vi "hse-configuration_GetAllKeysForSection.vi"(8 "error in (no error)":errorcluster, 10 "Section":string, 11 "hse-configuration in":refnum<class "hse-configuration.lvclass">) -> (0 "error out":errorcluster, 2 "Keys":string[](array[string]), 3 "hse-configuration out":refnum<class "hse-configuration.lvclass">)   [LabVIEW 2014, in "hse-configuration.lvclass"]
doc: "Reads the numeric configuration value (DOUBLE) identified by <b>section</b> and <b>key</b> from the configuration object\n\n____\nHAMPEL SOFTWARE ENGINEERING v0.12.0 (2018-09-13 18:21)"
uses:
  hse-configuration.lvclass
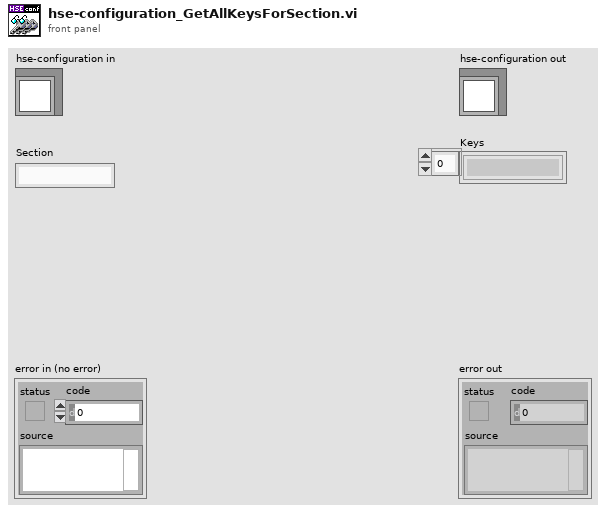
[diagram p1: front panel]
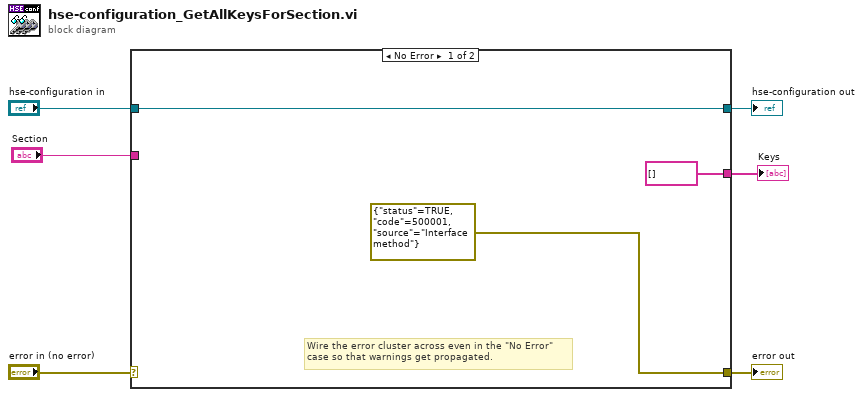
[diagram p0: block diagram]
diagram:
  n1 = case shown="No Error" "error in (no error)" {
    selector: "error in (no error)" -> [_ w11]
    tunnel: [errorcluster {"status"=TRUE, "code"=500001, "source"="Interface method"} ("error IO") w11] -> w5
    tunnel: [w9 w10] -> w3
    tunnel: "hse-configuration in" -> [w9 w10]
    tunnel: [string[] [] ("Sections") _] -> w2
    tunnel: "Section" -> [_ _]
    frame No Error {
      # "Wire the error cluster across even in the \"No Error\"\ncase so that warnings get propagated."
    }
    frame Error {
    }
  }
  "error out" <- w5
  "hse-configuration out" <- w3
  "Keys" <- w2
